vi "Set Cal Alert.vi"(8 "error IO":errorcluster, 10 "Calibration Alert?":bool, 11 "VISA resource name":refnum<visa-resource-name>) -> (0 "error Out":errorcluster, 3 "VISA resource Out":refnum<visa-resource-name>)   [LabVIEW 2012, in "Associated Research 78XX Series.lvlib"]
uses:
  <instrlib>/Associated Research 78XX Series/Associated Research 78XX Series.lvlib
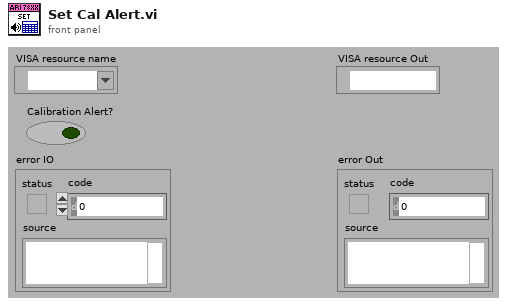
[diagram p1: front panel]
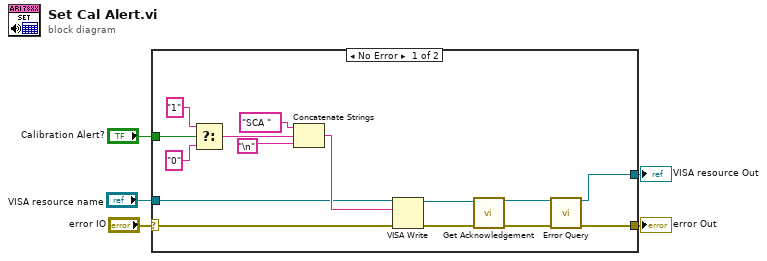
[diagram p0: block diagram]
diagram:
  n1 = case shown="No Error" "error IO" {
    selector: "error IO" -> [w20 w22]
    tunnel: [w18 w22] -> w2
    tunnel: [w19 w21] -> w3
    tunnel: "VISA resource name" -> [w7 w21]
    tunnel: "Calibration Alert?" -> [w9 _]
    frame No Error {
      n2 = Select(t="1", s=w9, f="0") -> (s? t:f=w10:string)
      n3 = Concatenate Strings("SCA " ("Command to Send (empty)"), w10, "\n") -> (w15:string)
      n4 = VISA Write(VISA resource name=w7, write buffer=w15, error in (no error)=w20) -> (VISA resource name out=w6:refnum<visa-resource-name>, error out=w8:errorcluster)  [unwired: 1 out]
      n5 = call <instrlib>:"Get Acknowledgement.vi"("VISA resource name"=w6, "error in (no error)"=w8) -> ("VISA resource name out"=w14:refnum<visa-resource-name>, "error out"=w13:errorcluster)  [unwired: 12 in]
      n6 = call <instrlib>:"Error Query.vi"("VISA resource name"=w14, "error in (no error)"=w13) -> ("VISA resource name out"=w19:refnum<visa-resource-name>, "error out"=w18:errorcluster)  [unwired: 10 in, 2 out]
    }
    frame Error {
    }
  }
  "VISA resource Out" <- w3
  "error Out" <- w2
